vi "Stop Core.vi"(10 "final error code":i32, 11 "LHW-GUI-Actor in":refnum<class "LHW-GUI-Actor.lvclass">) -> (3 "LHW-GUI-Actor out":refnum<class "LHW-GUI-Actor.lvclass">)   [LabVIEW 2016, in "LHW-GUI.lvlib" / "LHW-GUI-Actor.lvclass"]
doc: "(<B>Filename</B>: Actor Framework.lvlib:Actor.lvclass:Stop Core.vi)\n\nDefines what the actor does before it stops. Use the <B>final error code</B> input to determine whether the actor shut down in response to an error.\n\nBy default, this method does nothing. A descendant class may override it to define behavior, such as shutting down any processes the actor initiated in its override of the Actor Core method."
uses:
  LHW-GUI-Actor.lvclass
  <vilib>/event_ctls.llb/usereventprio.ctl
  LHW-GUI-Actor.lvclass/LHW-GUI-Actor.ctl
  <vilib>/ActorFramework/Actor/Actor.lvclass
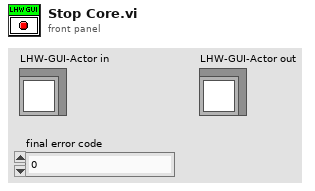
[diagram p1: front panel]
types:
  T1 = typedef "usereventprio.ctl" = enum32{"high priority", "normal priority"}
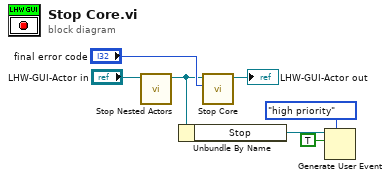
[diagram p0: block diagram]
diagram:
  n1 = call "Stop Nested Actors.vi"("LHW-GUI-Actor in"="LHW-GUI-Actor in") -> ("LHW-GUI-Actor out"=w1:refnum<class "LHW-GUI-Actor.lvclass">)  [unwired: 9 in, 1 out]
  n2 = Unbundle By Name(w1) -> ("Stop"=w5:refnum<user-event>)
  n3 = call-parent "Stop Core.vi"("final error code"="final error code", "Actor in"=w1) -> ("Actor out"=→"LHW-GUI-Actor out":refnum<class "LHW-GUI-Actor.lvclass">)  [unwired: 9 in]
  n4 = Generate User Event(priority (normal)=usereventprio."high priority", user event=w5, event data cluster=TRUE ("event data")) -> ()  [unwired: 1 in, 2 out]
